vi "Read Setup.vi"(8 "error in":errorcluster, 11 "File Path in":path) -> (0 "error out":errorcluster, 2 "Setup Data":T1={"DataBase Data"={"Api Token"="", "Organization"="", "url"="", "Organization ID"=""}, "Write Data"={"Bucket"="Test", "Timestamp precision"=enum."Seconds", "Line protocol"="", "Measurement"=""}, "Query - csv"=""}, 3 "File Path out":path)   [LabVIEW 2020, in "InfluxDB v2 Client.lvlib"]
doc: "Reads all settings for the test application from the setup file"
uses:
  InfluxDB v2 Client.lvlib
  Setup Data.ctl
  Client/DataBase Data.ctl
  Client/Write Data.ctl
  Client/Write Precision.ctl
  <vilib>/Utility/xml.llb/Read From XML File(string).vi
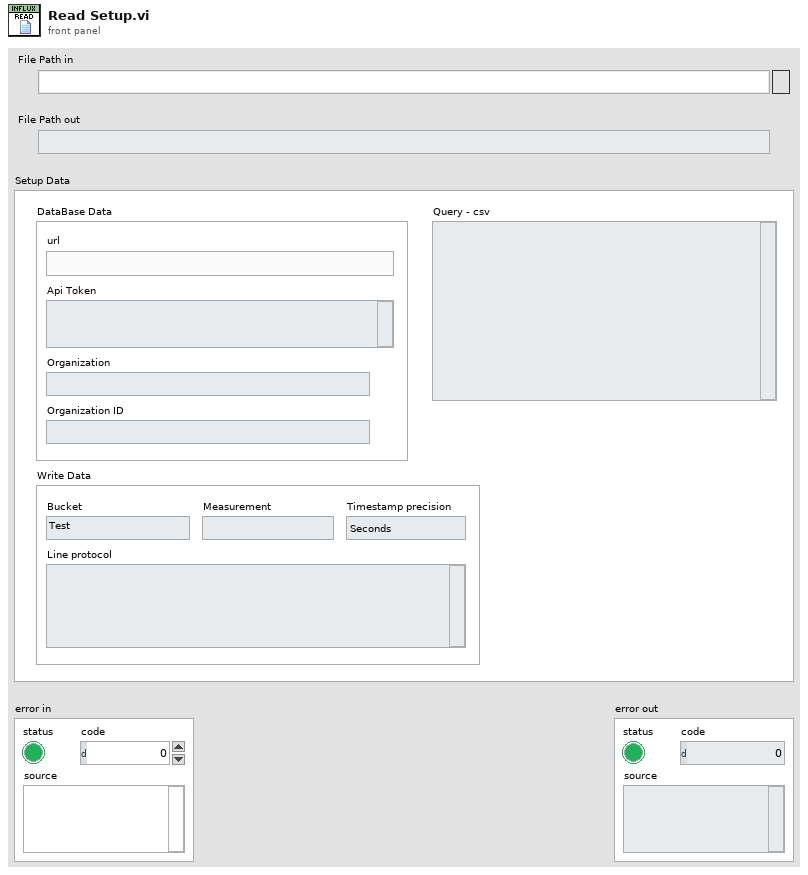
[diagram p1: front panel]
types:
  T1 = typedef "InfluxDB v2 Client.lvlib/Setup Data.ctl" = cluster{"DataBase Data":T2, "Write Data":T3, "Query - csv":string}
  T2 = typedef "InfluxDB v2 Client.lvlib/DataBase Data.ctl" = cluster{"Api Token":string, "Organization":string, "url":string, "Organization ID":string}
  T3 = typedef "InfluxDB v2 Client.lvlib/Write Data.ctl" = cluster{"Bucket":string, "Timestamp precision":T4, "Line protocol":string, "Measurement":string}
  T4 = typedef "InfluxDB v2 Client.lvlib/Write Precision.ctl" = enum16{"Nanoseconds", "Microseconds", "Milliseconds", "Seconds"}
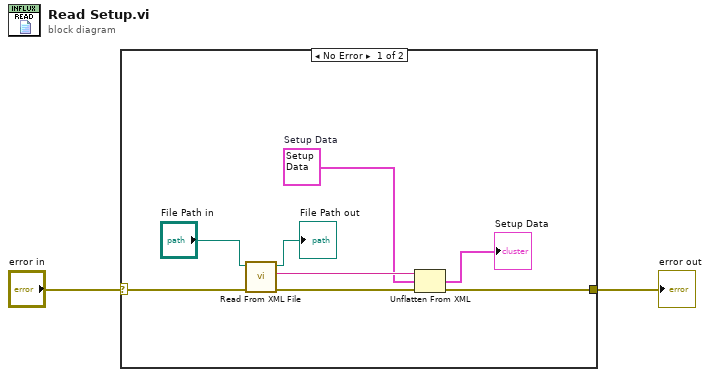
[diagram p0: block diagram]
diagram:
  n1 = case shown="No Error" "error in" {
    selector: "error in" -> [w10 w11]
    tunnel: [w5 w11] -> w1
    frame No Error {
      w6 = T1 {"DataBase Data"={"Api Token"="", "Organization"="", "url"="", "Organization ID"=""}, "Write Data"={"Bucket"="", "Timestamp precision"=enum."Seconds", "Line protocol"="", "Measurement"=""}, "Query - csv"=""}  # Setup Data
      n2 = call-poly <vilib>:"Read From XML File.vi"("error in (no error)"=w10, "XML File Path"="File Path in") -> ("error out"=w8:errorcluster, "XML Elements"=w7:string, "XML File Path(duplicate)"=→"File Path out":path)  [unwired: 7 in]
      n3 = Unflatten From XML(xml string=w7, type=w6, error in (no error)=w8) -> (value=→"Setup Data":T1, error out=w5:errorcluster)
    }
    frame Error {
    }
  }
  "error out" <- w1
